vi "ExOpenGlobalCam.vi"() -> ()   [LabVIEW 2010]
uses:
  CamHandle.vi
panel:
  out "Camera Opened":bool
  out "error out":errorcluster
  in  "error in (no error)":errorcluster
  # "ExOpenGlobalCam\nThis vi opens a camera and stores the handle in a global variable.\nThis vi MUST be run before any vi using the global camera handle."
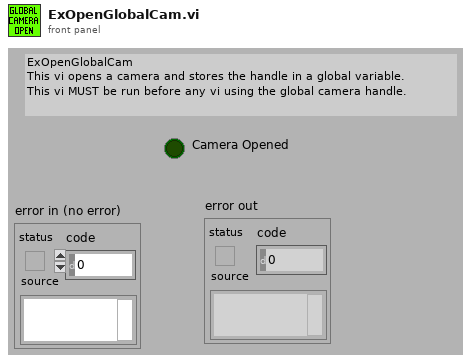
[diagram p1: front panel]
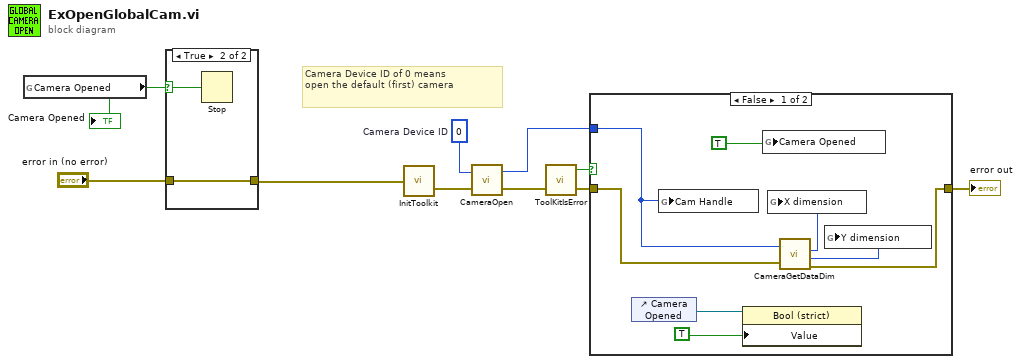
[diagram p0: block diagram]
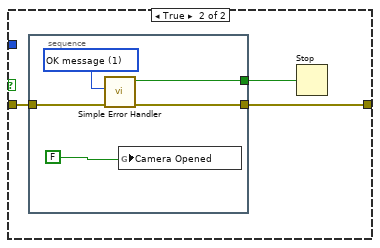
[diagram p3: hidden frame]
diagram:
  w6 = u32 0  # Camera Device ID
  # "Camera Device ID of 0 means\nopen the default (first) camera"
  n1 = global read "CamHandle.vi" "Camera Opened"() -> (w3:bool)
  "Camera Opened" <- w3
  n2 = case shown="True" w3 {
    selector: w3 -> [_ w12]
    tunnel: [w11 w13] -> w1
    tunnel: "error in (no error)" -> [w11 w13]
    frame False {
    }
    frame True {
      n3 = Stop(stop? (T)=w12) -> ()
    }
  }
  n4 = call <userlib>:"InitToolkit.vi"("error in"=w1) -> ("error out"=w10:errorcluster)
  n5 = call <userlib>:"CameraOpen.vi"("error in"=w10, "Camera Device ID"=w6) -> ("error out"=w9:errorcluster, "Camera Handle"=w5:u32)
  n6 = call <userlib>:"ToolKitIsError.vi"("error in"=w9) -> ("error out"=w7:errorcluster, "Error Flag"=w8:bool)  [unwired: 1 in]
  n7 = case shown="False" w8 {
    tunnel: w7 -> [w18 w24]
    tunnel: [w17 w23] -> w4
    tunnel: w5 -> [w19 _]
    frame False {
      n8 = control-ref of="Camera Opened"() -> (w14:refnum<vi>)
      n9 = global write "CamHandle.vi" "Cam Handle"(w19) -> ()
      n10 = property class="Bool (strict)"(reference=w14, "Value"=TRUE) -> ()  [unwired: 1 in, 2 out]
      n11 = global write "CamHandle.vi" "Camera Opened"(TRUE) -> ()
      n12 = call <userlib>:"CameraGetDataDim.vi"("Camera Handle"=w19, "error in"=w18) -> ("Xdim"=w21:u32, "Ydim"=w20:u32, "error out"=w17:errorcluster)  [unwired: 1 out]
      n13 = global write "CamHandle.vi" "X dimension"(w21) -> ()
      n14 = global write "CamHandle.vi" "Y dimension"(w20) -> ()
    }
    frame True {
      n15 = stacked-sequence {
        tunnel: w24 -> [w28]
        tunnel: [w27] -> w22
        tunnel: [w26] -> w23
        frame #0 {
          w29 = u16 1 items=["no dialog", "OK message", "continue or stop message"] ("type of dialog (OK msg:1)")
          n16 = call <vilib>:"Simple Error Handler.vi"("type of dialog (OK msg:1)"=w29, "error in (no error)"=w28) -> ("error?"=w27:bool, "error out"=w26:errorcluster)  [unwired: 3 in, 3 out]
          n17 = global write "CamHandle.vi" "Camera Opened"(FALSE) -> ()
        }
      }
      n18 = Stop(stop? (T)=w22) -> ()
    }
  }
  "error out" <- w4
